vi "p8.13.vi"() -> ()   [LabVIEW 2020]
uses:
  <vilib>/vision/NI_Vision_Development_Module.lvlib
panel:
  in  "Kernel":sgl[][](array[numeric])=[[1.0, 1.0, 1.0, 0.0], [1.0, 1.0, 1.0, 0.0], [1.0, 1.0, 1.0, 0.0], [0.0, 0.0, 0.0, 1.0]] format="%.2f"
  out "imagen filtrada":T1(plugin-control)
  out "imagen suma":T1(plugin-control)
  out "Imagen k=20":T1(plugin-control)
  in  "k2":dbl=20.0 format="%#_13g"
  out "Imagen k=2":T1(plugin-control)
  in  "k1":dbl=2.0 format="%#_13g"
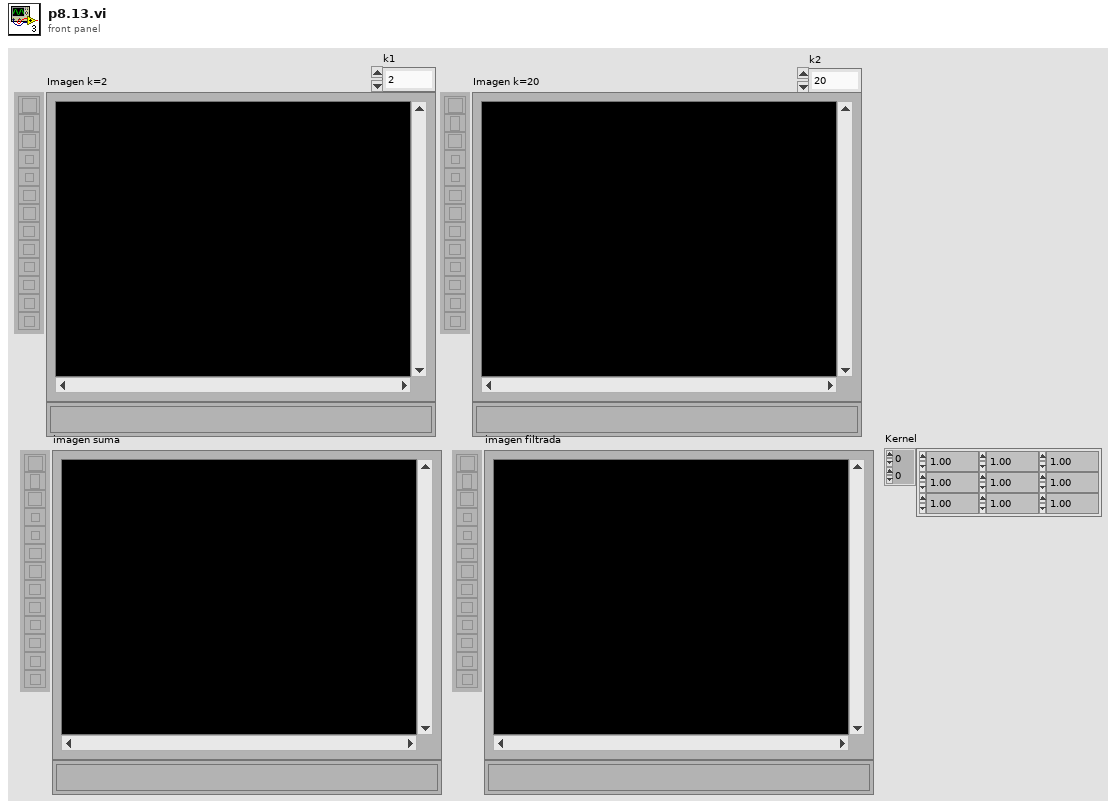
[diagram p1: front panel]
types:
  T1 = typedef "IMAQ Image.ctl" = refnum<image>
  T2 = typedef "Image Type" = u32
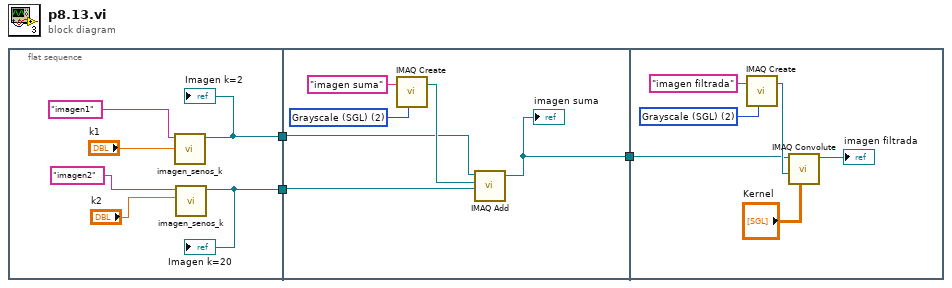
[diagram p0: block diagram]
diagram:
  n1 = flat-sequence {
    tunnel: [w5] -> w3
    tunnel: [w4] -> w2
    tunnel: w3 -> [w12]
    tunnel: w2 -> [w11]
    tunnel: [w10] -> w1
    tunnel: w1 -> [w17]
    frame #0 {
      n2 = call "imagen_senos_k.vi"("k"="k1", "Image Name"="imagen1") -> ("Imagen"=w5:T1)  [unwired: 9 in]
      "Imagen k=2" <- w5
      n3 = call "imagen_senos_k.vi"("k"="k2", "Image Name"="imagen2") -> ("Imagen"=w4:T1)  [unwired: 9 in]
      "Imagen k=20" <- w4
    }
    frame #1 {
      w13 = T2 2 items=["Grayscale (U8)", "Grayscale (I16)", "Grayscale (SGL)", "Complex (CSG)", "RGB (U32)", "HSL (U32)", "RGB (U64)", "Grayscale (U16)"] ("Image Type")
      n4 = call "IMAQ Create"("Image Name"="imagen suma", "Image Type"=w13) -> ("New Image"=w15:T1)  [unwired: 3 in, 1 out]
      n5 = call "IMAQ Add"("Image Src A"=w12, "Image Dst"=w15, "Image Src B"=w11) -> ("Image Dst Out"=w10:T1)  [unwired: 4 in, 1 out]
      "imagen suma" <- w10
    }
    frame #2 {
      w21 = T2 2 items=["Grayscale (U8)", "Grayscale (I16)", "Grayscale (SGL)", "Complex (CSG)", "RGB (U32)", "HSL (U32)", "RGB (U64)", "Grayscale (U16)"] ("Image Type")
      n6 = call "IMAQ Create"("Image Name"="imagen filtrada", "Image Type"=w21) -> ("New Image"=w19:T1)  [unwired: 3 in, 1 out]
      n7 = call "IMAQ Convolute"("Kernel"="Kernel", "Image Dst"=w19, "Image Src"=w17) -> ("Image Dst Out"=→"imagen filtrada":T1)  [unwired: 7 in, 1 out]
    }
  }
